vi "Configure Serial Bus (UART - Trigger).vi"(0 "VISA resource name":refnum<visa-resource-name>, 1 "Burst Value (1 pulses)":dbl=1.0, 2 "Data Thresholds (0)":i32, 5 "Serial Bus Name (1: Serial Bus 1)":i32(ring)=1 items=["Serial Bus 1"=1, "Serial Bus 2"=2], 7 "Trigger Type (0: Receive Start)":i32(ring) items=["Receive Start", "Receive Stop", "Receive Data", "RD1", "RD0", "RDx", "Parity Error", "Transmit Start", "Transmit Stop", "Transmit Data", "TD1", "TD0", "TDx"], 9 "Enable Burst (F: Disable)":bool, 11 "error in (no error)":errorcluster, 12 "Burst Idle Period (0.005 S)":dbl=0.005, 13 "Qualifier (0: Equal)":i32(ring) items=["Equal", "Not Equal", "Greater Than", "Less Than"]) -> (4 "VISA resource name out":refnum<visa-resource-name>, 15 "error out":errorcluster)   [LabVIEW 2023, in "Keysight-DSQx3014T.lvlib"]
doc: "Configures the trigger settings of UART bus."
uses:
  Keysight-DSQx3014T.lvlib
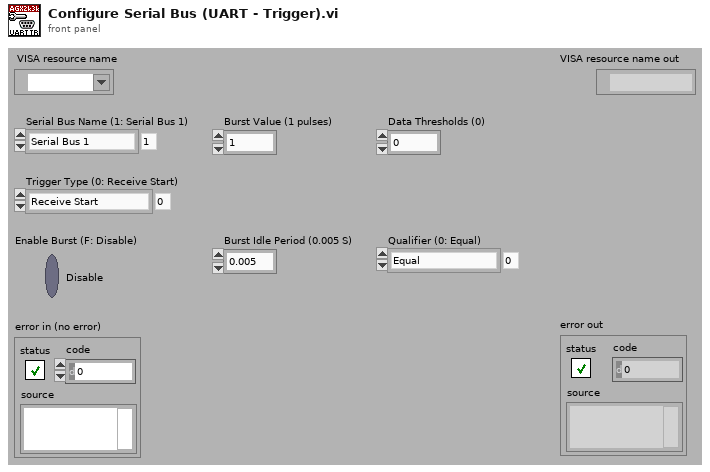
[diagram p1: front panel]
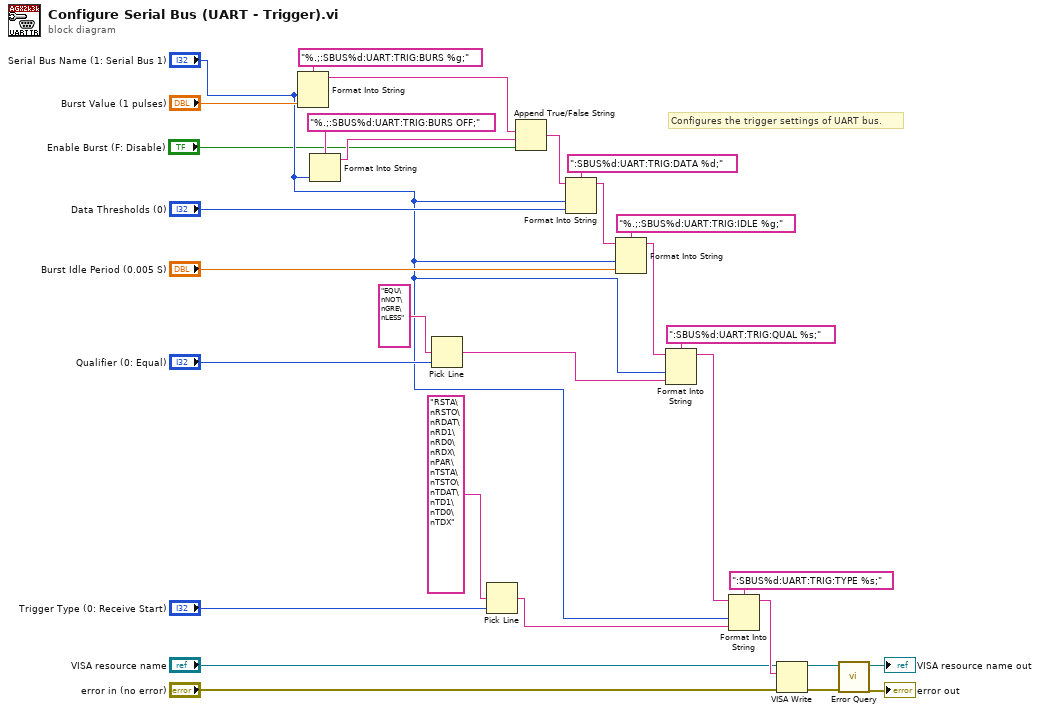
[diagram p0: block diagram]
diagram:
  # "Configures the trigger settings of UART bus."
  n1 = Format Into String(format string="%.;:SBUS%d:UART:TRIG:BURS %g;", "Serial Bus Name (1: Serial Bus 1)", "Burst Value (1 pulses)") -> (resulting string=w3:string)  [unwired: 2 in, 1 out]
  n2 = Format Into String(format string="%.;:SBUS%d:UART:TRIG:BURS OFF;", "Serial Bus Name (1: Serial Bus 1)") -> (resulting string=w4:string)  [unwired: 2 in, 1 out]
  n3 = Pick Line(multi-line string="EQU\nNOT\nGRE\nLESS", line index="Qualifier (0: Equal)") -> (output string=w19:string)  [unwired: 1 out]
  n4 = Pick Line(multi-line string="RSTA\nRSTO\nRDAT\nRD1\nRD0\nRDX\nPAR\nTSTA\nTSTO\nTDAT\nTD1\nTD0\nTDX", line index="Trigger Type (0: Receive Start)") -> (output string=w14:string)  [unwired: 1 out]
  n5 = Append True/False String(1:"Enable Burst (F: Disable)", 2:w4, 3:w3) -> (0:w2:string)  [unwired: 1 out]
  n6 = Format Into String(format string=":SBUS%d:UART:TRIG:DATA %d;", initial string=w2, "Serial Bus Name (1: Serial Bus 1)", "Data Thresholds (0)") -> (resulting string=w26:string)  [unwired: 1 in, 1 out]
  n7 = Format Into String(format string="%.;:SBUS%d:UART:TRIG:IDLE %g;", initial string=w26, "Serial Bus Name (1: Serial Bus 1)", "Burst Idle Period (0.005 S)") -> (resulting string=w21:string)  [unwired: 1 in, 1 out]
  n8 = Format Into String(format string=":SBUS%d:UART:TRIG:QUAL %s;", initial string=w21, "Serial Bus Name (1: Serial Bus 1)", w19) -> (resulting string=w16:string)  [unwired: 1 in, 1 out]
  n9 = Format Into String(format string=":SBUS%d:UART:TRIG:TYPE %s;", initial string=w16, "Serial Bus Name (1: Serial Bus 1)", w14) -> (resulting string=w13:string)  [unwired: 1 in, 1 out]
  n10 = VISA Write(VISA resource name="VISA resource name", write buffer=w13, error in (no error)="error in (no error)") -> (VISA resource name out=w10:refnum<visa-resource-name>, error out=w9:errorcluster)  [unwired: 1 out]
  n11 = call "Error Query.vi"("error in (no error)"=w9, "VISA resource name"=w10) -> ("error out"=→"error out":errorcluster, "VISA resource name out"=→"VISA resource name out":refnum<visa-resource-name>)  [unwired: 8 out]
